vi "Write File Ref+.vi"(8 "error in (no error)":errorcluster, 10 "File Ref":refnum<file>, 11 "File Handler in":refnum<class "File Handler.lvclass">) -> (0 "error out":errorcluster, 3 "File Handler out":refnum<class "File Handler.lvclass">)   [LabVIEW 2018, in "GLog.lvlib" / "File Handler.lvclass"]
uses:
  File Handler.lvclass
  File Handler.lvclass/File Handler.ctl
  RolloverTrigger/RolloverTrigger.lvclass
panel:
  # "Connector Pane"
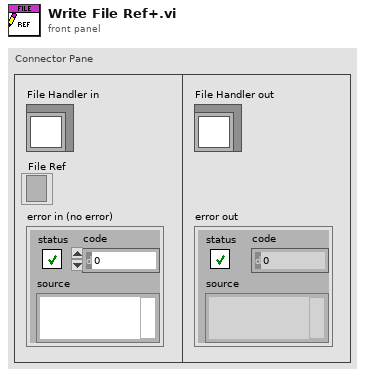
[diagram p1: front panel]
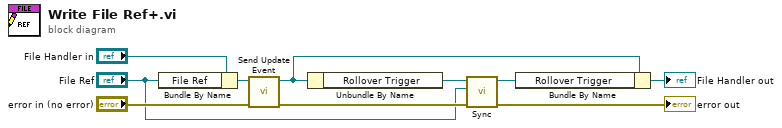
[diagram p0: block diagram]
diagram:
  n1 = Bundle By Name(cluster="File Handler in", "File Ref"="File Ref") -> (w8:refnum<class "File Handler.lvclass">)
  n2 = call "Send Update Event.vi"("error in (no error)"="error in (no error)", "File Handler in"=w8) -> ("error out"=w3:errorcluster, "File Handler out"=w5:refnum<class "File Handler.lvclass">)  [unwired: 8 in]
  n3 = Unbundle By Name(w5) -> ("Rollover Trigger"=w7:refnum<class "RolloverTrigger.lvclass">)
  n4 = call-dynamic "Sync.vi"("error in (no error)"=w3, "file ref"="File Ref", "rollover trigger in"=w7) -> ("error out"=→"error out":errorcluster, "rollover trigger out"=w6:refnum<class "RolloverTrigger.lvclass">)  [unwired: 7 in]
  n5 = Bundle By Name(cluster=w5, "Rollover Trigger"=w6) -> (→"File Handler out":refnum<class "File Handler.lvclass">)
